vi "FTW-Ether-Destroy.vi"(5 "Force Destroy?":bool, 11 "error in":errorcluster) -> (15 "error out":errorcluster)   [LabVIEW 2012, in "FTW-Actor.lvlib" / "FTW-Ether.lvclass"]
uses:
  FTW-Ether.lvclass
  EventLogger/FTW-Logger.lvclass
  FTW-Ether-Instance.vi
panel:
  # "Inputs"
  # "Outputs"
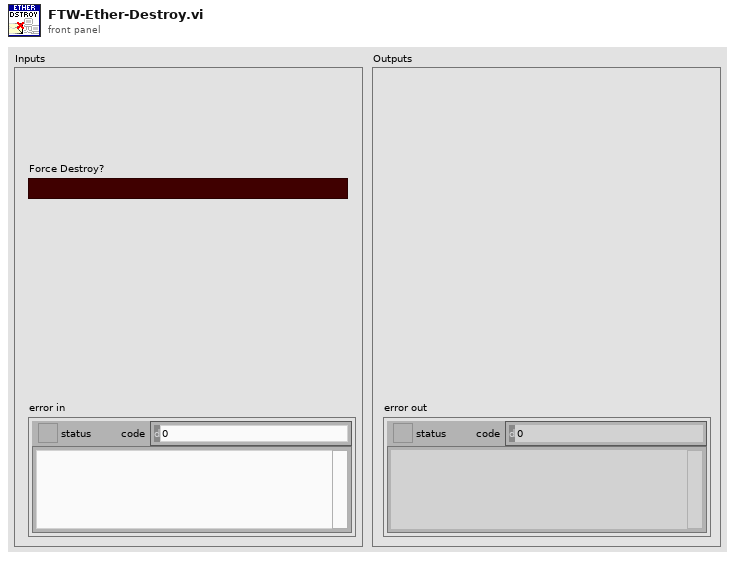
[diagram p1: front panel]
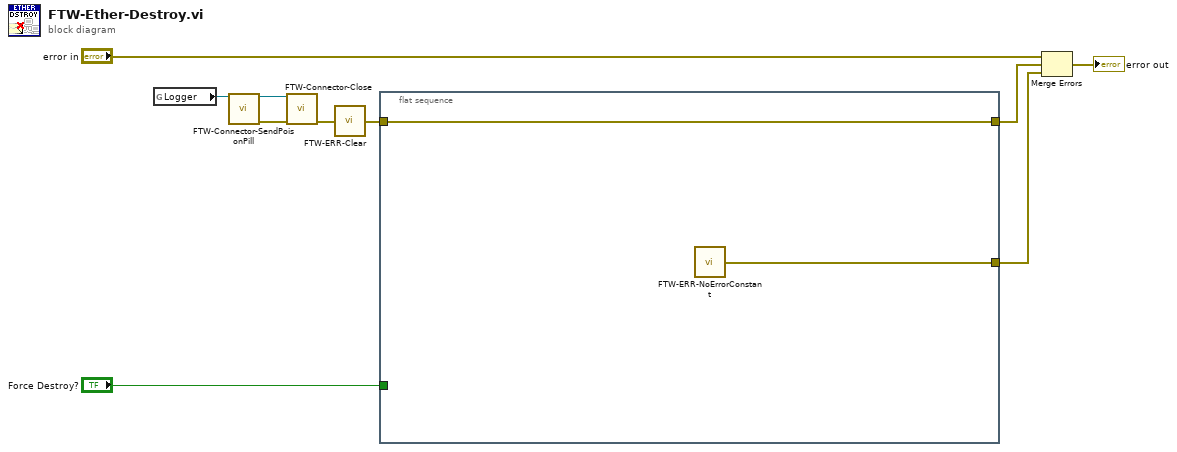
[diagram p0: block diagram]
diagram:
  n1 = global read "FTW-Ether-Instance.vi" "Logger"() -> (w1:refnum<class "FTW-Logger.lvclass">)
  n2 = call-dynamic "FTW-Connector-SendPoisonPill.vi"("FTW Actor Connector"=w1) -> ("FTW Actor Connector out"=w8:refnum<class "FTW-Logger.lvclass">, "error out"=w7:errorcluster)  [unwired: 10 in, 3 out]
  n3 = call-dynamic "FTW-Connector-Close.vi"("FTW Actor Connector"=w8, "error in"=w7) -> ("error out"=w3:errorcluster)  [unwired: 13 in]
  n4 = call "FTW-ERR-Clear.vi"("error to snuff"=w3) -> ("no error"=w2:errorcluster)
  n5 = flat-sequence {
    tunnel: "Force Destroy?" -> [_]
    tunnel: w2 -> [w12]
    tunnel: [w12] -> w5
    tunnel: [w11] -> w4
    frame #0 {
      n6 = call "FTW-ERR-NoErrorConstant.vi"() -> ("no error"=w11:errorcluster)
    }
  }
  n7 = Merge Errors("error in", w5, w4) -> (→"error out":errorcluster)
